vi "Register Collector.vi"(8 "error in (no error)":errorcluster, 10 "Collector":refnum<class "Collectable.lvclass">, 11 "Session Handle in":T1) -> (0 "error out":errorcluster, 3 "Session Handle out":T1)   [LabVIEW 2020, in "Registry.lvlib" / "Registry Session.lvclass"]
uses:
  Registry Session.lvclass
  Typedefs/Session Handle.ctl
  collector/collectable/Collectable.lvclass
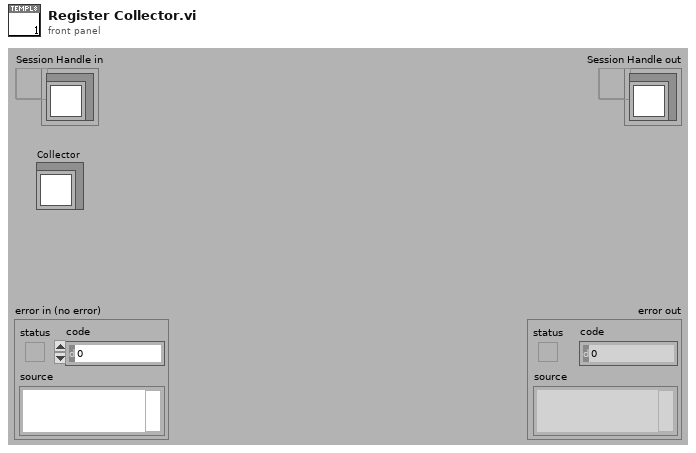
[diagram p1: front panel]
types:
  T1 = typedef "Registry.lvlib/Registry Session.lvclass/Session Handle.ctl" = refnum<data-value>
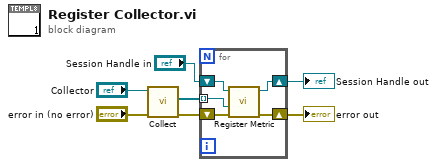
[diagram p0: block diagram]
diagram:
  n1 = call-dynamic "Collect.vi"("error in (no error)"="error in (no error)", "Collectable in"="Collector") -> ("error out"=w3:errorcluster, "Metrics"=w2:refnum<data-value>[])  [unwired: 7 in, 1 out]
  n2 = for {
    shift-right: [w11] -> w4
    shift-left: "Session Handle in" -> [w12]
    shift-right: [w8] -> w1
    shift-left: w3 -> [w10]
    tunnel: w2 -> [w9] mode=indexing
    n3 = call "Register Metric.vi"("error in (no error)"=w10, "New Metric"=w9, "Session Handle in"=w12) -> ("error out"=w8:errorcluster, "Session Handle out"=w11:T1)  [unwired: 7 in]
  }
  "Session Handle out" <- w4
  "error out" <- w1
